vi "MSScript_Format_LinearAmpScan.vi"(9 "ValueArray":string[](array[string]), 10 "NameArray":string[](array[string]), 11 "MSScript in":refnum<class "MSScript.lvclass">) -> (0 "ValueErrorArray":bool[](array[boolean]), 1 "TagErrorArray":bool[](array[boolean]), 2 "ParamErrorArray":bool[](array[boolean]), 3 "data out":variant, 4 "#ofParamError":bool)   [LabVIEW 2018, in "MSScript.lvclass"]
uses:
  MSScript.lvclass
  Ctl/MSEditorParam ampScan.ctl
  MSScript.lvclass/MSScript.ctl
  MSScript_Transform_UInt.vi
  MSScript_Transform_Extended.vi
  MSScript_Transform_EXTArray.vi
  MSScript_Transform_Boolean.vi
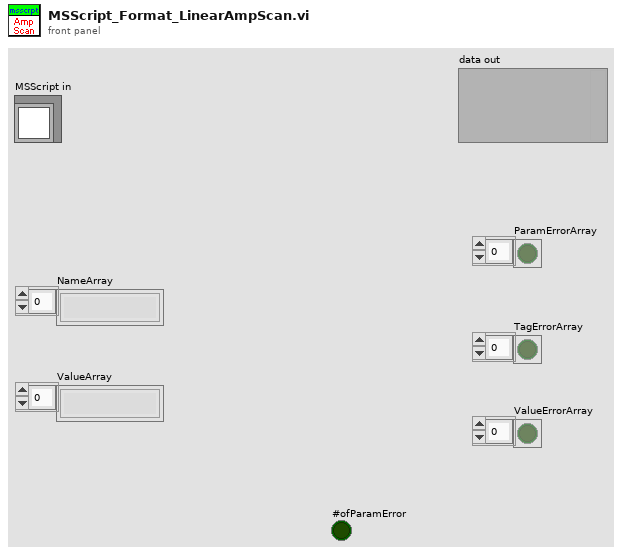
[diagram p1: front panel]
types:
  T1 = typedef "MSEditorParam ampScan.ctl" = cluster{"AuxWfmType":u32, "iAuxCyc":ext, "Beta":ext, "BetaScale":ext, "AuxAmp":ext[], "AuxPulse1":ext[], "AuxPulse2":ext[], "AuxPulseAmp":ext[], "Time":ext, "Amp":ext[], "Continuous":bool}
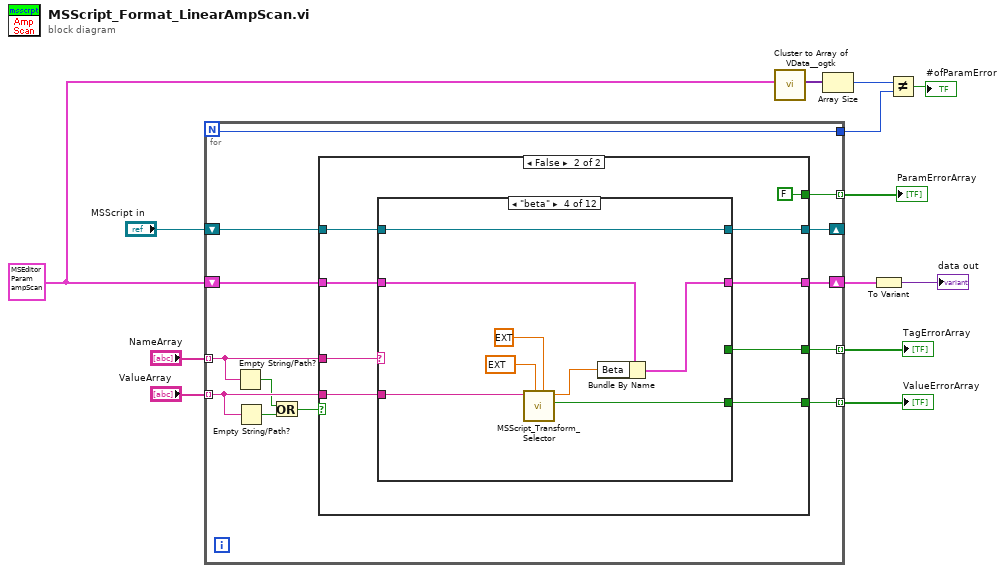
[diagram p0: block diagram]
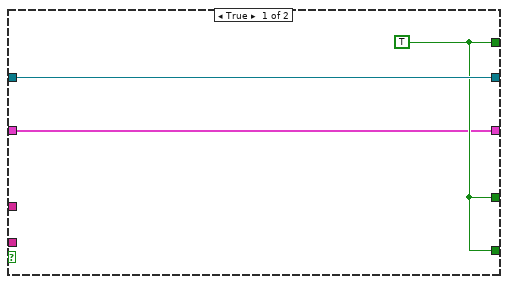
[diagram p2: hidden frame]
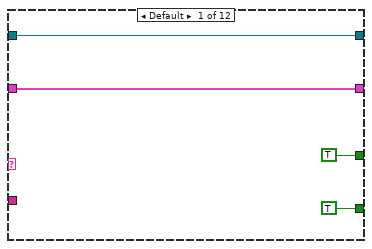
[diagram p3: hidden frame]
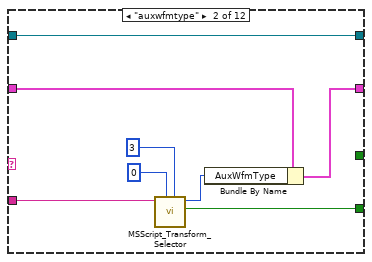
[diagram p4: hidden frame]
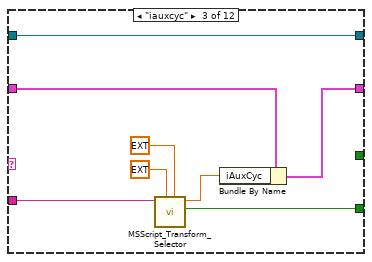
[diagram p5: hidden frame]
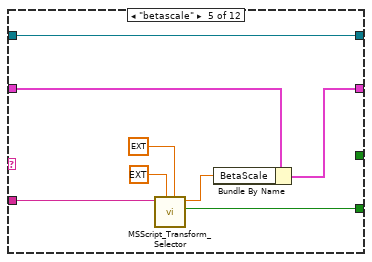
[diagram p6: hidden frame]
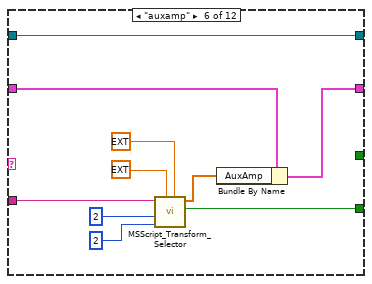
[diagram p7: hidden frame]
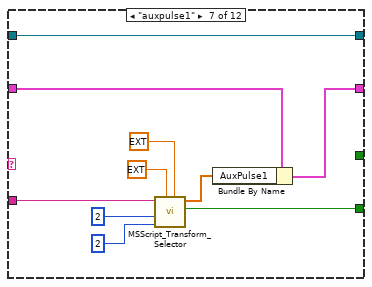
[diagram p8: hidden frame]
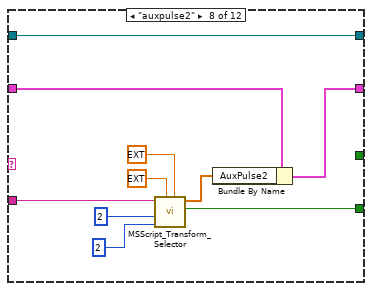
[diagram p9: hidden frame]
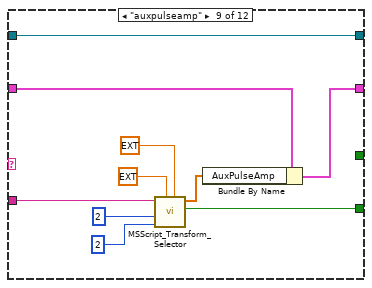
[diagram p10: hidden frame]
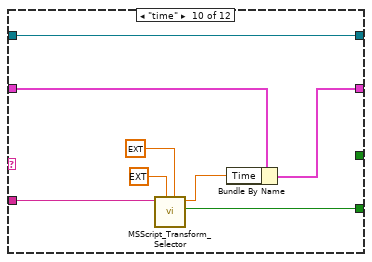
[diagram p11: hidden frame]
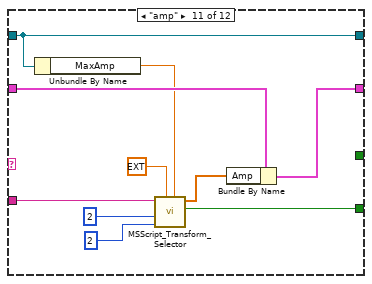
[diagram p12: hidden frame]
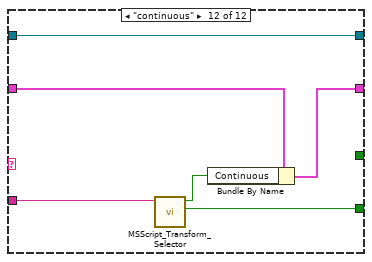
[diagram p13: hidden frame]
diagram:
  w8 = T1 {"AuxWfmType"=0, "iAuxCyc"=0.0, "Beta"=0.5, "BetaScale"=1.0, "AuxAmp"=[], "AuxPulse1"=[0.0, 0.5], "AuxPulse2"=[0.5, 0.99], "AuxPulseAmp"=[1.0, -1.0], "Time"=1.0, "Amp"=[200.0, 300.0], "Continuous"=FALSE} ("ParamValueType")
  n1 = for {
    N -> [w14]
    tunnel: "NameArray" -> [w22] mode=indexing
    tunnel: "ValueArray" -> [w21] mode=indexing
    tunnel: [w26] -> w13 mode=indexing
    tunnel: [w24] -> w12 mode=indexing
    tunnel: [w17] -> w11 mode=indexing
    shift-right: [w15] -> w9
    shift-left: w8 -> [w16]
    tunnel: [w14] -> w4
    shift-right: [w23] -> _
    shift-left: "MSScript in" -> [w25]
    n2 = Empty String/Path?(string/path=w22) -> (empty?=w19:bool)
    n3 = Empty String/Path?(string/path=w21) -> (empty?=w20:bool)
    n4 = Or(x=w19, y=w20) -> (x .or. y?=w18:bool)
    n5 = case shown="False" w18 {
      tunnel: [w28 w32] -> w26
      tunnel: w25 -> [w29 w37]
      tunnel: [w28 w33] -> w24
      tunnel: [w29 w30] -> w23
      tunnel: w22 -> [_ w35]
      tunnel: w21 -> [_ w34]
      tunnel: [w28 FALSE] -> w17
      tunnel: w16 -> [w27 w36]
      tunnel: [w27 w31] -> w15
      frame True {
        w28 = TRUE
      }
      frame False {
        n6 = case shown="\"beta\"" w35 {
          tunnel: [TRUE _ _ _ _ _ _ _ _ _ _ _] -> w32
          tunnel: w37 -> [w40 w48 w56 w64 w72 w82 w92 w102 w112 w120 w126 w134]
          tunnel: w34 -> [_ w49 w57 w65 w73 w83 w93 w103 w113 w121 w131 w137]
          tunnel: [TRUE ("Value Error?") w50 w58 w66 w74 w84 w94 w104 w114 w122 w132 w138] -> w33
          tunnel: [w40 w48 w56 w64 w72 w82 w92 w102 w112 w120 w126 w134] -> w30
          tunnel: w36 -> [w39 w46 w54 w62 w70 w81 w90 w100 w110 w118 w129 w136]
          tunnel: [w39 w45 w53 w61 w69 w80 w89 w99 w109 w117 w128 w135] -> w31
          frame Default {
          }
          frame "auxwfmtype" {
            n7 = call-poly "MSScript_Transform_Selector.vi"("upper limit"=u64 3, "lower limit"=u64 0, "string in"=w49) -> ("Value Error?"=w50:bool, "Value Output"=w47:u64)  [unwired: 6 in, 1 out]
            n8 = Bundle By Name(cluster=w46, "AuxWfmType"=w47) -> (w45:T1)
          }
          frame "iauxcyc" {
            n9 = call-poly "MSScript_Transform_Selector.vi"("upper limit (Inf)"=ext 1.0 ("upper limit"), "lower limit (-Inf)"=ext 0.0 ("lower limit"), "Check_Str"=w57) -> ("Value Error?"=w58:bool, "Value Output"=w55:ext)  [unwired: 6 in, 1 out]
            n10 = Bundle By Name(cluster=w54, "iAuxCyc"=w55) -> (w53:T1)
          }
          frame "beta" {
            n11 = call-poly "MSScript_Transform_Selector.vi"("upper limit (Inf)"=ext 1.0 ("upper limit"), "lower limit (-Inf)"=ext 0.01 ("lower limit"), "Check_Str"=w65) -> ("Value Error?"=w66:bool, "Value Output"=w63:ext)  [unwired: 6 in, 1 out]
            n12 = Bundle By Name(cluster=w62, "Beta"=w63) -> (w61:T1)
          }
          frame "betascale" {
            n13 = call-poly "MSScript_Transform_Selector.vi"("upper limit (Inf)"=ext 10.0 ("upper limit"), "lower limit (-Inf)"=ext 0.0 ("lower limit"), "Check_Str"=w73) -> ("Value Error?"=w74:bool, "Value Output"=w71:ext)  [unwired: 6 in, 1 out]
            n14 = Bundle By Name(cluster=w70, "BetaScale"=w71) -> (w69:T1)
          }
          frame "auxamp" {
            n15 = call-poly "MSScript_Transform_Selector.vi"("upper limit (Inf)"=ext 1.0 ("upper limit"), "lower limit (-Inf)"=ext 0.0 ("lower limit"), "MinSize"=u8 2, "MaxSize"=u8 2, "check_str"=w83) -> ("Value Error?"=w84:bool, "Value Output"=w75:ext[])  [unwired: 4 in, 1 out]
            n16 = Bundle By Name(cluster=w81, "AuxAmp"=w75) -> (w80:T1)
          }
          frame "auxpulse1" {
            n17 = call-poly "MSScript_Transform_Selector.vi"("upper limit (Inf)"=ext 1.0 ("upper limit"), "lower limit (-Inf)"=ext 0.0 ("lower limit"), "MinSize"=u8 2 ("MaxSize"), "MaxSize"=u8 2, "check_str"=w93) -> ("Value Error?"=w94:bool, "Value Output"=w91:ext[])  [unwired: 4 in, 1 out]
            n18 = Bundle By Name(cluster=w90, "AuxPulse1"=w91) -> (w89:T1)
          }
          frame "auxpulse2" {
            n19 = call-poly "MSScript_Transform_Selector.vi"("upper limit (Inf)"=ext 1.0 ("upper limit"), "lower limit (-Inf)"=ext 0.0 ("lower limit"), "MinSize"=u8 2 ("MaxSize"), "MaxSize"=u8 2, "check_str"=w103) -> ("Value Error?"=w104:bool, "Value Output"=w101:ext[])  [unwired: 4 in, 1 out]
            n20 = Bundle By Name(cluster=w100, "AuxPulse2"=w101) -> (w99:T1)
          }
          frame "auxpulseamp" {
            n21 = call-poly "MSScript_Transform_Selector.vi"("upper limit (Inf)"=ext 1.0 ("upper limit"), "lower limit (-Inf)"=ext -1.0 ("lower limit"), "MinSize"=u8 2 ("MaxSize"), "MaxSize"=u8 2, "check_str"=w113) -> ("Value Error?"=w114:bool, "Value Output"=w111:ext[])  [unwired: 4 in, 1 out]
            n22 = Bundle By Name(cluster=w110, "AuxPulseAmp"=w111) -> (w109:T1)
          }
          frame "time" {
            n23 = call-poly "MSScript_Transform_Selector.vi"("upper limit (Inf)"=ext 50.0 ("upper limit"), "lower limit (-Inf)"=ext 0.0 ("lower limit"), "Check_Str"=w121) -> ("Value Error?"=w122:bool, "Value Output"=w119:ext)  [unwired: 6 in, 1 out]
            n24 = Bundle By Name(cluster=w118, "Time"=w119) -> (w117:T1)
          }
          frame "amp" {
            n25 = Unbundle By Name(w126) -> ("MaxAmp"=w125:ext)
            n26 = call-poly "MSScript_Transform_Selector.vi"("upper limit (Inf)"=w125, "lower limit (-Inf)"=ext 0.0 ("lower limit"), "MinSize"=2 ("MaxSize"), "MaxSize"=2, "check_str"=w131) -> ("Value Error?"=w132:bool, "Value Output"=w130:ext[])  [unwired: 4 in, 1 out]
            n27 = Bundle By Name(cluster=w129, "Amp"=w130) -> (w128:T1)
          }
          frame "continuous" {
            n28 = call-poly "MSScript_Transform_Selector.vi"("Check_Str"=w137) -> ("Value Error?"=w138:bool, "Value Output"=w133:bool)  [unwired: 9 in]
            n29 = Bundle By Name(cluster=w136, "Continuous"=w133) -> (w135:T1)
          }
        }
      }
    }
  }
  "TagErrorArray" <- w13
  "ValueErrorArray" <- w12
  "ParamErrorArray" <- w11
  n30 = call <userlib>:"Cluster to Array of VData__ogtk.vi"("Cluster"=w8) -> ("Array of VData"=w7:variant[])  [unwired: 9 in, 1 out]
  n31 = Array Size(array=w7) -> (size(s)=w3:i32)
  n32 = To Variant(anything=w9) -> (Variant=→"data out":variant)
  n33 = Not Equal?(x=w3, y=w4) -> (x != y?=→"#ofParamError":bool)
